vi "3DClassificationDisplay.vi"(8 "error in":errorcluster, 11 "Parameter":T1={"3D Plot"=[], "3D Scatter"=refnum, "Data"={"Split"={"X Train"=[], "X Test"=[], "Y Train"=[], "Y Test"=[]}, "Predict"=[]}, "Display"={"Choice"=enum."All", "Indexe"={"X"=0, "Y"=1, "Z"=2}}, "Point Property"={"Train Style"=enum."Full circle", "Test OK Style"=enum."Full square", "Label Color"=[8978528, 4367871, 1985280], "Test NO OK"={"Style"=enum."Cross", "Color"=16716800}}, "3D Plot Datatype.lvclass"=refnum}) -> (0 "error out":errorcluster)   [LabVIEW 2020]
doc: "Displays the trained or tested data in 3D"
uses:
  _Controls/3DParameters.ctl
  <vilib>/Math Plots/3D Math Plots/3D Plot/3D Plot Datatype/3D Plot Datatype.lvclass
  <vilib>/Math Plots/3D Math Plots/3D Scatter/3D Scatter XCtrl/3D Scatter.xctl
  _Controls/Datas.ctl
  _Controls/PointPropertyMultipleLabel.ctl
  _Controls/Style.ctl
  _Controls/3DData.ctl
panel:
  in  "Local":T6={"Parameter"={"3D Plot"=[], "3D Scatter"=refnum, "Data"={"Split"={"X Train"=[], "X Test"=[], "Y Train"=[], "Y Test"=[]}, "Predict"=[]}, "Display"={"Choice"=enum."All", "Indexe"={"X"=0, "Y"=1, "Z"=2}}, "Point Property"={"Train Style"=enum."Full circle", "Test OK Style"=enum."Full square", "Label Color"=[8978528, 4367871, 1985280], "Test NO OK"={"Style"=enum."Cross", "Color"=16716800}}, "3D Plot Datatype.lvclass"=refnum}, "3DArray"=[], "Rating 3D Array"=[], "GoodPredict"=0, "Point ID"=[]}
types:
  T1 = typedef "3DParameters.ctl" = cluster{"3D Plot":refnum<class "3D Plot Datatype.lvclass">[], "3D Scatter":refnum<vi>, "Data":T2, "Display":cluster{"Choice":enum16{"All", "Train", "Test"}, "Indexe":cluster{"X":i32, "Y":i32, "Z":i32}}, "Point Property":T3, "3D Plot Datatype.lvclass":refnum<class "3D Plot Datatype.lvclass">}
  T2 = typedef "Datas.ctl" = cluster{"Split":cluster{"X Train":dbl[][], "X Test":dbl[][], "Y Train":dbl[][], "Y Test":dbl[][]}, "Predict":dbl[][]}
  T3 = typedef "PointPropertyMultipleLabel.ctl" = cluster{"Train Style":T4, "Test OK Style":T4, "Label Color":u32[], "Test NO OK":cluster{"Style":T4, "Color":u32}}
  T4 = typedef "Style.ctl" = enum16{"Empty circle", "Full circle", "Empty square", "Full square", "Cross"}
  T5 = typedef "3DData.ctl" = cluster{"Tag":i32, "X":dbl[], "Y":dbl[], "Z":dbl[]}
  T6 = cluster{"Parameter":T1, "3DArray":cluster{"X":dbl[], "Y":dbl[], "Z":dbl[]}[], "Rating 3D Array":T5[], "GoodPredict":i32, "Point ID":cluster{"DataUse":enum16{"Dataset", "Train", "Test"}, "Color":u32}[]}
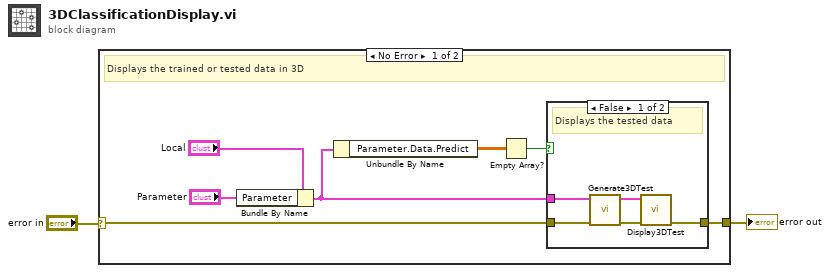
[diagram p0: block diagram]
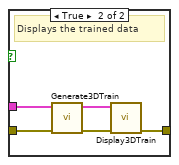
[diagram p2: hidden frame]
diagram:
  n1 = case shown="No Error" "error in" {
    selector: "error in" -> [w5 w20]
    tunnel: [w4 w20] -> w1
    frame No Error {
      # "Displays the trained or tested data in 3D"
      n2 = Bundle By Name(cluster="Local", "Parameter"="Parameter") -> (w3:T6)
      n3 = Unbundle By Name(w3) -> ("Parameter.Data.Predict"=w7:dbl[][])
      n4 = Empty Array?(array=w7) -> (empty?=w6:bool)
      n5 = case shown="False" w6 {
        tunnel: w5 -> [w14 w19]
        tunnel: [w10 w17] -> w4
        tunnel: w3 -> [w13 w15]
        frame False {
          # "Displays the tested data"
          n6 = call "Generate3DTest.vi"("error in (no error)"=w14, "Local"=w13) -> ("error out"=w11:errorcluster, "Local Out"=w12:T6)  [unwired: 8 in]
          n7 = call "Display3DTest.vi"("error in"=w11, "Local"=w12) -> ("error out"=w10:errorcluster)  [unwired: 8 in, 1 out]
        }
        frame True {
          # "Displays the trained data"
          n8 = call "Generate3DTrain.vi"("error in"=w19, "Local"=w15) -> ("error out"=w18:errorcluster, "Local Out"=w16:T6)  [unwired: 8 in]
          n9 = call "Display3DTrain.vi"("error in"=w18, "Local"=w16) -> ("error out"=w17:errorcluster)  [unwired: 8 in, 1 out]
        }
      }
    }
    frame Error {
    }
  }
  "error out" <- w1
